vi "AK-LNI COM Init.vi"(9 "TimeOut (ms)":u32=10000, 11 "Schnittstelle":T1={"VISA resource name"="COM1", "baud rate"=38400, "data bits"=8, "parity"=0, "stop bits"=10, "flow control"=0} {"flow control" items=["None"=0, "XON/XOFF"=1, "RTS/CTS"=2, "DTR/DSR"=4]; "stop bits" items=["1.0"=10, "1.5"=15, "2.0"=20]; "parity" items=["None", "Odd", "Even", "Mark", "Space"]; "data bits" min=5 max=8 step=1}) -> (0 "error out":errorcluster caption="Fehler (Ausgang)", 3 "VISA resource name":refnum<visa-resource-name> caption="VISA-Ressourcenname (Ausgang)")   [LabVIEW 2020, in "Linearisierung v2.lvlib" / "Gasteiler.lvlib" / "AK Komm Gasteiler.lvlib"]
doc: "Das Telegrammformat sieht nach jeder Nachricht das ASCII-Steuerzeichen ETX vor. Die COM-Schnittstelle muss daher das Abschlußzeichen aktivieren und als Endzeichen ETX (\\03 = 0x03) verwenden. Das Anfordern von N Bytes wird so entweder nach dem Lesen von ETX oder nach dem Einlangen von N Zeichen beendet. Die Zahl N wird so hoch gewählt, dass alle Antworten durch ETX beendet werden.\n\nDie Parameter sind fest eingestellt auf 9600 Baud, 8N1. Das Messgerät verwendet RTS/CTS nicht. Die Einstellung am Messgerät sind abzustimmen."
uses:
  AK Komm Gasteiler.lvlib
  AK-Schnittstelle/Serielle Parameter.ctl
  <vilib>/Instr/_visa.llb/VISA Configure Serial Port (Instr).vi
  AK-Schnittstelle/AK Seriell/AK Seriell.lvlib
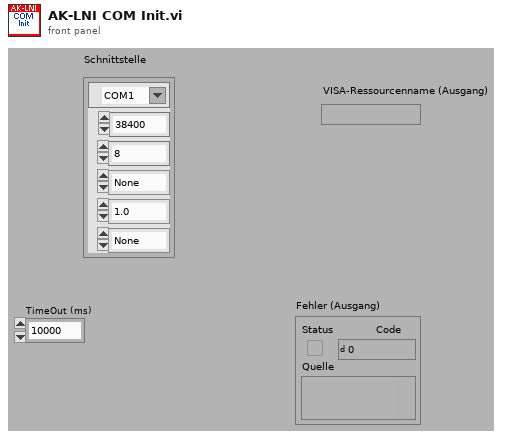
[diagram p1: front panel]
types:
  T1 = typedef "AK-Schnittstelle.lvlib/AK Seriell.lvlib/Serielle Parameter.ctl" = cluster{"VISA resource name":refnum<visa-resource-name>, "baud rate":u32, "data bits":u16, "parity":u16, "stop bits":u16, "flow control":u16}
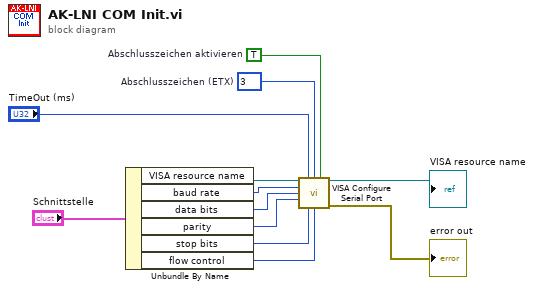
[diagram p0: block diagram]
diagram:
  w11 = TRUE  # Abschlusszeichen aktivieren
  w12 = u8 3  # Abschlusszeichen (ETX)
  n1 = Unbundle By Name("Schnittstelle") -> ("VISA resource name"=w6:refnum<visa-resource-name>, "baud rate"=w5:u32, "data bits"=w4:u16, "parity"=w3:u16, "stop bits"=w2:u16, "flow control"=w1:u16)
  n2 = call-poly "VISA Configure Serial Port"("VISA resource name"=w6, "timeout (10sec)"="TimeOut (ms)", "termination char\n(0xA = '\\n' = LF)"=w12, "Enable Termination\nChar (T)"=w11, "baud rate (9600)"=w5, "data bits (8)"=w4, "parity (0:none)"=w3, "stop bits (10: 1 bit)"=w2, "flow control (0:none)"=w1) -> ("VISA resource name out"=→"VISA resource name":refnum<visa-resource-name>, "error out"=→"error out":errorcluster)  [unwired: 5 in]
